vi "Read Array of VacuumLine Objs.vi"(11 "VacuumLines in":refnum<class "VacuumLines.lvclass">) -> (2 "Array of VacuumLine Objs":refnum<class "VacuumLine.lvclass">[](array[class]), 3 "VacuumLines out":refnum<class "VacuumLines.lvclass">)   [LabVIEW 2016, in "Hardware.lvlib" / "VacuumLine.lvlib" / "VacuumLines.lvclass"]
uses:
  <userlib>/Common Components/Hardware/Abstract System/VacuumLine/VacuumLines/VacuumLines.lvclass
  <userlib>/Common Components/Hardware/Abstract System/VacuumLine/VacuumLine/VacuumLine.lvclass
  <userlib>/Common Components/Hardware/Abstract System/VacuumLine/VacuumLines/VacuumLines.lvclass/VacuumLines.ctl
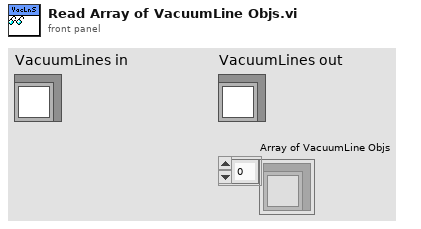
[diagram p1: front panel]
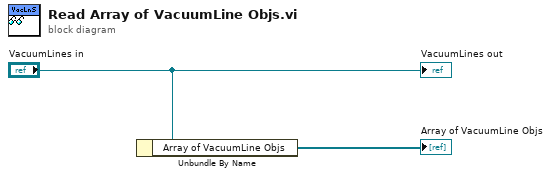
[diagram p0: block diagram]
diagram:
  n1 = Unbundle By Name("VacuumLines in") -> ("Array of VacuumLine Objs"=→"Array of VacuumLine Objs":refnum<class "VacuumLine.lvclass">[])
  "VacuumLines out" <- "VacuumLines in"
